vi "傅里叶基矢 6.vi"() -> ()   [LabVIEW 2016]
panel:
  out "Numeric":i32
  out "base":dbl[][](graph)
  out "show":dbl[][](graph)
  out "read":u32[][](graph)
  in  "path to JPEG file":path
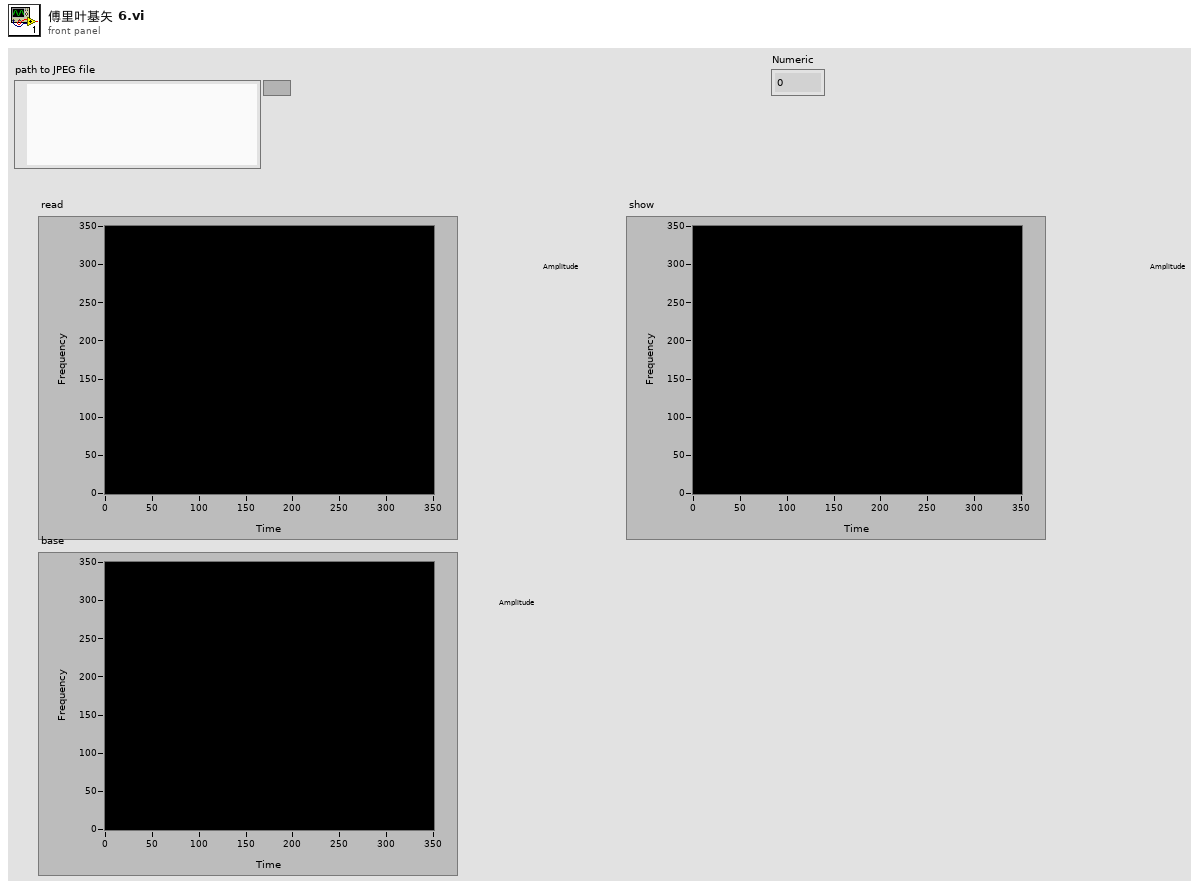
[diagram p1: front panel]
types:
  T1 = typedef "imagedata.ctl" = cluster{"image type":i32, "image depth":i32, "image":u8[], "mask":u8[], "colors":u32[], "Rectangle":cluster{"left":i16, "top":i16, "right":i16, "bottom":i16}}
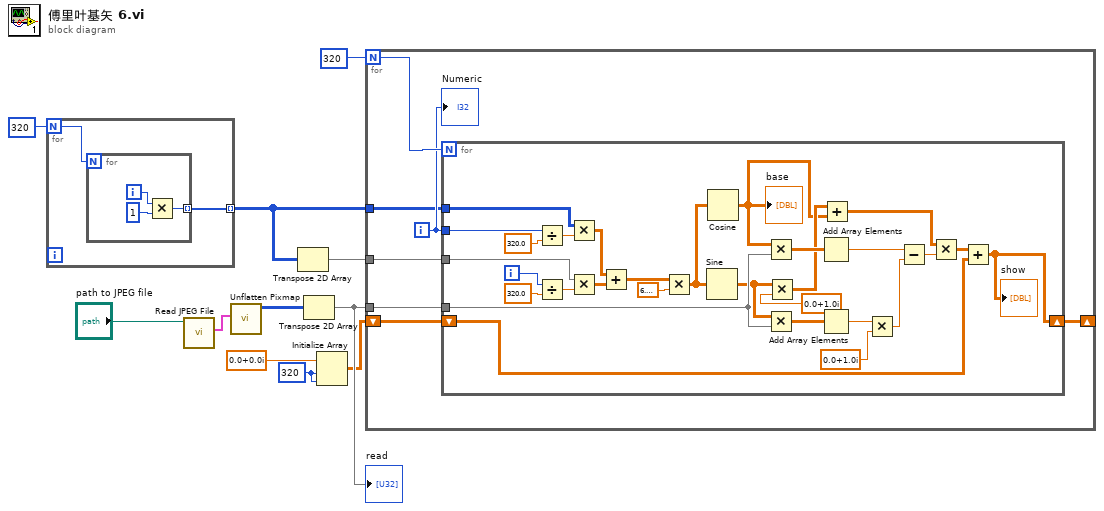
[diagram p0: block diagram]
diagram:
  w1 = 320 ("dimension size")
  n1 = for {
    N: 320 -> [w13]
    tunnel: [w12] -> w5 mode=indexing
    n2 = for {
      N: w13 -> [_]
      tunnel: [w14] -> w12 mode=indexing
      i -> [w16]
      n3 = Multiply(x=w16, y=1) -> (x*y=w14:i32)
    }
  }
  n4 = call <vilib>:"Read JPEG File.vi"("path to JPEG file"="path to JPEG file") -> ("image data"=w11:T1)  [unwired: 8 in, 2 out]
  n5 = call <vilib>:"Unflatten Pixmap.vi"("image data"=w11) -> ("24-bit pixmap"=w9:u32[][])  [unwired: 4 in, 6 out]
  n6 = Transpose 2D Array(2D array=w5) -> (transposed array=w6:i32[][])
  n7 = Transpose 2D Array(2D array=w9) -> (transposed array=w4:u32[][])
  "read" <- w4
  n8 = Initialize Array(cdb 0.0+0.0i ("element"), w1, w1) -> (w3:cdb[][])
  n9 = for {
    N: 320 -> [w23]
    tunnel: w6 -> [w22]
    tunnel: w5 -> [w20]
    tunnel: w4 -> [w19]
    shift-right: [w17] -> _
    shift-left: w3 -> [w18]
    i -> [w21]
    n10 = for {
      N: w23 -> [_]
      tunnel: w22 -> [w48]
      tunnel: w21 -> [w47]
      tunnel: w20 -> [w45]
      tunnel: w19 -> [w40]
      shift-right: [w28] -> w17
      shift-left: w18 -> [w29]
      i -> [w50]
      n11 = Divide(x=w47, y=320.0) -> (x/y=w46:dbl)
      n12 = Divide(x=w50, y=320.0) -> (x/y=w49:dbl)
      n13 = Multiply(x=w45, y=w46) -> (x*y=w44:dbl[][])
      n14 = Multiply(x=w48, y=w49) -> (x*y=w43:dbl[][])
      n15 = Add(x=w44, y=w43) -> (x+y=w42:dbl[][])
      n16 = Multiply(x=w42, y=6.283185307179586) -> (x*y=w35:dbl[][])
      n17 = Sine(x=w35) -> (sin(x)=w24:dbl[][])
      n18 = Cosine(x=w35) -> (cos(x)=w27:dbl[][])
      "base" <- w27
      n19 = Multiply(x=w27, y=w40) -> (x*y=w39:dbl[][])
      n20 = Multiply(x=w24, y=w40) -> (x*y=w38:dbl[][])
      n21 = Multiply(x=w24, y=cdb 0.0+1.0i) -> (x*y=w33:cdb[][])
      n22 = Add Array Elements(numeric array=w39) -> (sum=w26:dbl)
      n23 = Add Array Elements(numeric array=w38) -> (sum=w25:dbl)
      n24 = Add(x=w33, y=w27) -> (x+y=w32:cdb[][])
      n25 = Multiply(x=w25, y=cdb 0.0+1.0i) -> (x*y=w36:cdb)
      n26 = Subtract(x=w26, y=w36) -> (x-y=w31:cdb)
      n27 = Multiply(x=w32, y=w31) -> (x*y=w30:cdb[][])
      n28 = Add(x=w30, y=w29) -> (x+y=w28:cdb[][])
      "show" <- w28
    }
    "Numeric" <- w21
  }
